vi "Attachment.vi"(1 "Filename":path) -> (0 "Output String":string)   [LabVIEW 2010]
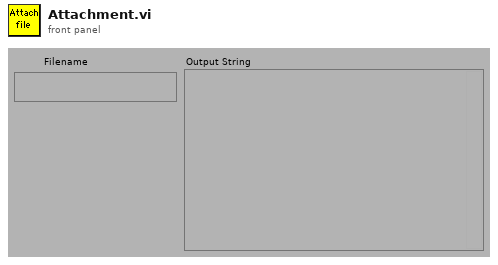
[diagram p1: front panel]
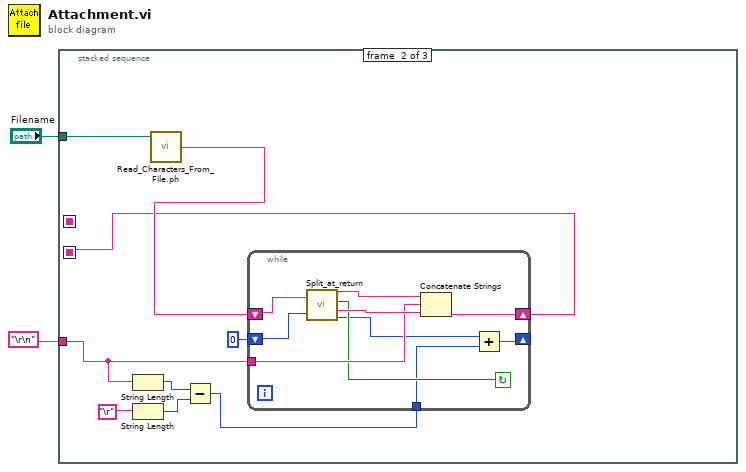
[diagram p0: block diagram]
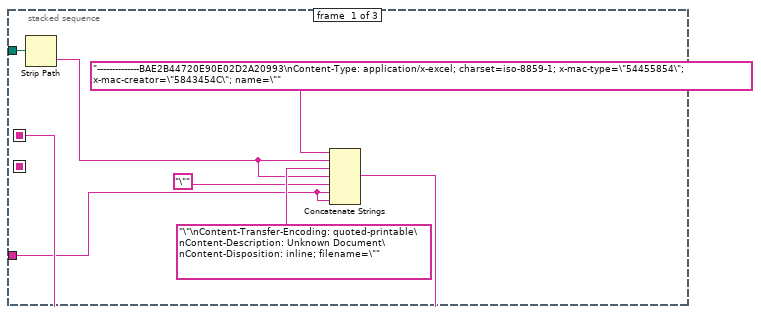
[diagram p2: hidden frame]
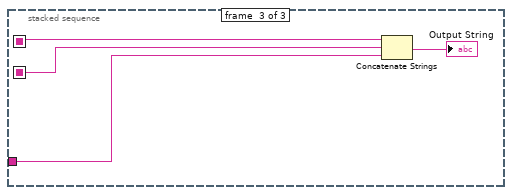
[diagram p3: hidden frame]
diagram:
  n1 = stacked-sequence {
    seq-local: [w6 _ _] -> [_ _ w32]
    seq-local: [_ w16 _] -> [_ _ w29]
    tunnel: "Filename" -> [w4 w15 _]
    tunnel: "\r\n" -> [w5 w13 w31]
    frame #0 {
      n2 = Strip Path(path=w4) -> (name=w3:string)  [unwired: 1 out]
      n3 = Concatenate Strings("--------------BAE2B44720E90E02D2A20993\nContent-Type: application/x-excel; charset=iso-8859-1; x-mac-type=\"54455854\"; x-mac-creator=\"5843454C\"; name=\"", w3, "\"\nContent-Transfer-Encoding: quoted-printable\nContent-Description: Unknown Document\nContent-Disposition: inline; filename=\"", w3, "\"", w5, w5) -> (w6:string)
    }
    frame #1 {
      n4 = String Length(string=w13) -> (length=w12:i32)
      n5 = String Length(string="\r") -> (length=w11:i32)
      n6 = call "Read_Characters_From_File.ph.vi"("file path (dialog if empty)"=w15) -> ("character string"=w18:string)  [unwired: 5 in, 3 out]
      n7 = Subtract(x=w12, y=w11) -> (x-y=w10:i32)
      n8 = while {
        tunnel: w10 -> [w19]
        shift-left: 0 ("offset past match") -> [w23]
        shift-right: [w20] -> _
        shift-left: w18 -> [w24]
        shift-right: [w25] -> w16
        tunnel: w13 -> [w26]
        stop <- w22 continue-if-true
        n9 = call "Split_at_return.vi"("String"=w24, "offset (0)"=w23) -> ("before substring"=w28:string, "Matched?"=w22:bool, "after substring"=w27:string, "offset past match"=w21:i32)
        n10 = Concatenate Strings(w28, w26, w27) -> (w25:string)
        n11 = Add(x=w21, y=w19) -> (x+y=w20:i32)
      }
    }
    frame #2 {
      n12 = Concatenate Strings(w32, w29, w31) -> (→"Output String":string)
    }
  }
